vi "PressureDrop.vi"() -> ()   [LabVIEW 2019]
uses:
  <vilib>/DAQmx/write.llb/DAQmx Write (Analog DBL 1Chan 1Samp).vi
  <vilib>/DAQmx/create/channels.llb/DAQmx Create Channel (AO-Voltage-Basic).vi
  <vilib>/DAQmx/miscellaneous.llb/DAQmx Fill In Error Info.vi
panel:
  in  "stop 2":bool
  in  "Flow Rate":dbl format="%0.2f"
  in  "NI Device":tag
  in  "stop":bool
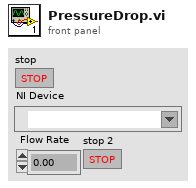
[diagram p1: front panel]
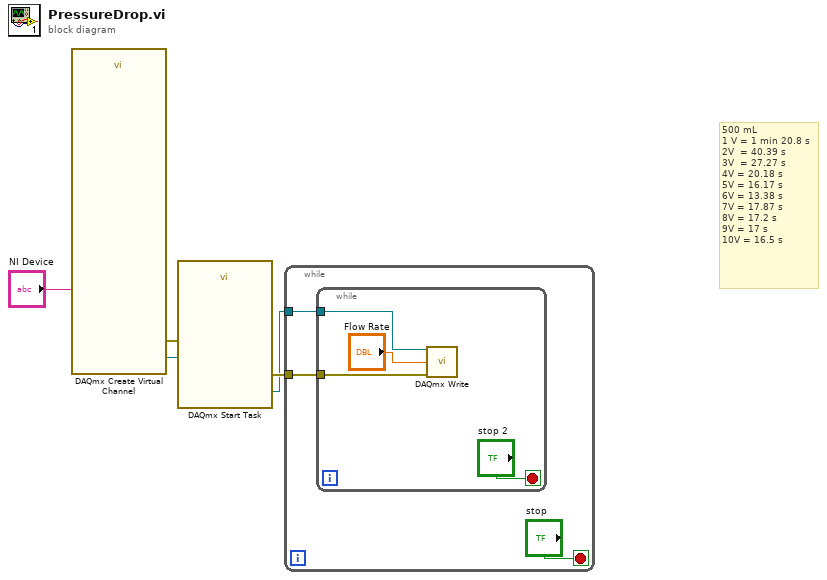
[diagram p0: block diagram]
diagram:
  # "500 mL\n1 V = 1 min 20.8 s \n2V  = 40.39 s \n3V  = 27.27 s\n4V = 20.18 s \n5V = 16.17 s\n6V = 13.38 s\n7V = 17.87 s\n8V = 17.2 s \n9V = 17 s\n10V = 16.5 s"
  n1 = call-poly <vilib>:"DAQmx Create Virtual Channel.vi"("physical channels"="NI Device") -> ("task out"=w5:refnum<k21>, "error out"=w4:errorcluster)  [unwired: 13 in]
  n2 = call <vilib>:"DAQmx Start Task.vi"("task/channels in"=w5, "error in"=w4) -> ("task out"=w1:refnum<k21>, "error out"=w2:errorcluster)  [unwired: 12 in]
  n3 = while {
    tunnel: w2 -> [w7]
    tunnel: w1 -> [w6]
    stop <- "stop" stop-if-true
    n4 = while {
      tunnel: w7 -> [w12]
      tunnel: w6 -> [w11]
      stop <- "stop 2" stop-if-true
      n5 = call-poly <vilib>:"DAQmx Write.vi"("task/channels in"=w11, "data"="Flow Rate", "error in"=w12) -> ()  [unwired: 10 in, 3 out]
    }
  }
